vi "RSZVB Read Limit Line Segment List.vi"(0 "VISA session":refnum<visa-resource-name>, 5 "Channel (Trace) (1)":i32=1, 11 "error in (no error)":errorcluster {"code" format="%.0x"}) -> (2 "Stop Response":dbl[](array[numeric]) format="%^.3e", 3 "Stop Stimulus":dbl[](array[numeric]) format="%^.3e", 4 "dup VISA session":refnum<visa-resource-name>, 6 "Start Stimulus":dbl[](array[numeric]) format="%^.3e", 8 "Segments Count":i32, 10 "Type":i32[](array[numeric]), 14 "Start Response":dbl[](array[numeric]) format="%^.3e", 15 "error out":errorcluster {"code" format="%.0x"})   [LabVIEW 2011]
doc: "This VI returns entire limit line segment list. The limit line segment is calculated as a straight line connecting the two points (<Start Stimulus>, <Start Response>) and (<Stop Stimulus>, <Stop Response>).\n\nRemote-control command(s):\nCALCulate<Ch/Tr>:LIMit:DATA?"
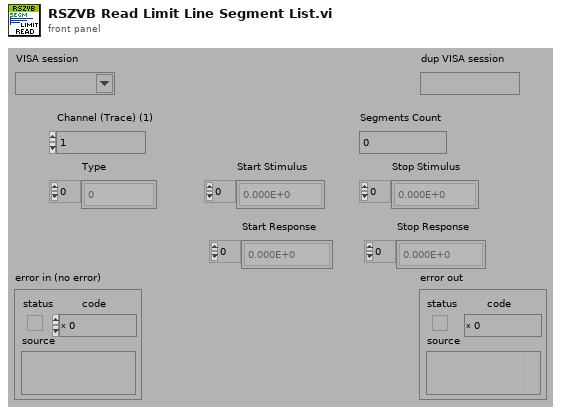
[diagram p1: front panel]
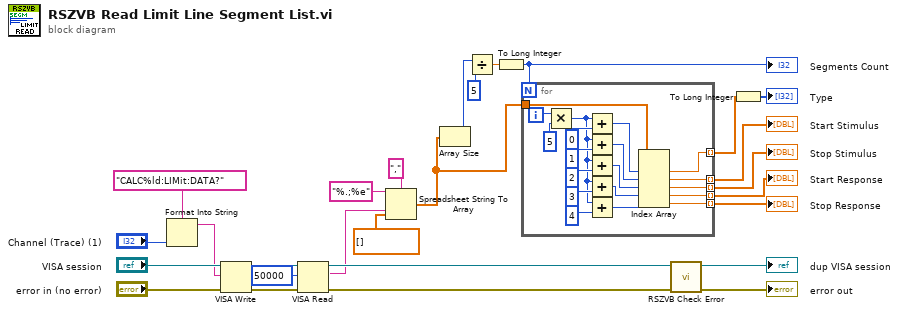
[diagram p0: block diagram]
diagram:
  n1 = Format Into String(format string="CALC%ld:LIMit:DATA?", "Channel (Trace) (1)") -> (resulting string=w18:string)  [unwired: 2 in, 1 out]
  n2 = VISA Write(VISA resource name="VISA session", write buffer=w18, error in (no error)="error in (no error)") -> (VISA resource name out=w27:refnum<visa-resource-name>, error out=w23:errorcluster)  [unwired: 1 out]
  n3 = VISA Read(VISA resource name=w27, byte count=u32 50000 ("byte count (0)"), error in (no error)=w23) -> (VISA resource name out=w25:refnum<visa-resource-name>, read buffer=w4:string, error out=w24:errorcluster)  [unwired: 1 out]
  n4 = Spreadsheet String To Array(delimiter (Tab)=",", format string="%.;%e", spreadsheet string=w4, array type (2D Dbl)=dbl[] []) -> (array=w5:dbl[])
  n5 = Array Size(array=w5) -> (size(s)=w6:i32)
  n6 = Divide(x=w6, y=5) -> (x/y=w3:dbl)
  n7 = To Long Integer(number=w3) -> (32bit integer=w2:i32)
  "Segments Count" <- w2
  n8 = for {
    N: w2 -> [_]
    tunnel: [w46] -> w11 mode=indexing
    tunnel: [w45] -> w10 mode=indexing
    tunnel: [w44] -> w9 mode=indexing
    tunnel: [w43] -> w8 mode=indexing
    tunnel: [w42] -> w7 mode=indexing
    tunnel: w5 -> [w32]
    i -> [w30]
    n9 = Multiply(x=w30, y=5) -> (x*y=w29:i32)
    n10 = Add(x=w29, y=0) -> (x+y=w33:i32)
    n11 = Add(x=w29, y=1) -> (x+y=w34:i32)
    n12 = Add(x=w29, y=2) -> (x+y=w35:i32)
    n13 = Add(x=w29, y=3) -> (x+y=w36:i32)
    n14 = Add(x=w29, y=4) -> (x+y=w37:i32)
    n15 = Index Array(array=w32, index #1=w33, index #2=w34, index #3=w35, index #4=w36, index #5=w37) -> (element #1=w46:dbl, element #2=w45:dbl, element #3=w44:dbl, element #4=w43:dbl, element #5=w42:dbl)
  }
  "Start Stimulus" <- w10
  "Stop Stimulus" <- w9
  "Start Response" <- w8
  "Stop Response" <- w7
  n16 = call "RSZVB Check Error.vi"("error in (no error)"=w24, "VISA session"=w25) -> ("error out"=→"error out":errorcluster, "dup VISA session"=→"dup VISA session":refnum<visa-resource-name>)  [unwired: 8 in]
  n17 = To Long Integer(number=w11) -> (32bit integer=→"Type":i32[])
